vi "add filepath.vi"(6 "priority (F)":bool, 8 "error in (no error)":errorcluster, 10 "filepath":path, 11 "ComicVine_manager in":refnum<class "ComicVine_manager.lvclass">) -> (0 "error out":errorcluster, 3 "ComicVine_manager out":refnum<class "ComicVine_manager.lvclass">)   [LabVIEW 2024, in "ComicVine_manager.lvclass"]
uses:
  ComicVine_manager.lvclass
  ComicVine_manager.lvclass/ComicVine_manager.ctl
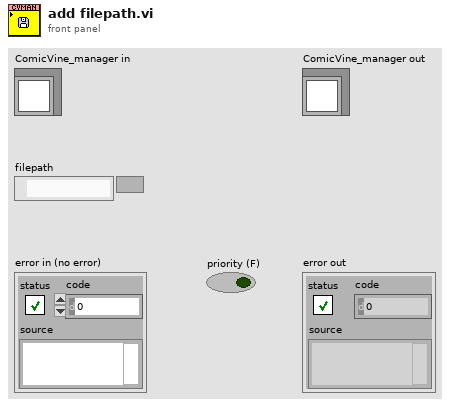
[diagram p1: front panel]
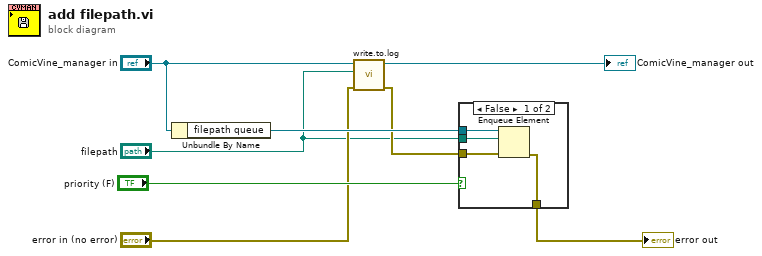
[diagram p0: block diagram]
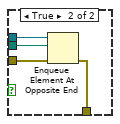
[diagram p2: hidden frame]
diagram:
  n1 = Unbundle By Name("ComicVine_manager in") -> ("filepath queue"=w8:refnum<queue>)
  n2 = call "write.to.log"("error in (no error)"="error in (no error)", "new path"="filepath", "ComicVine_manager in"="ComicVine_manager in") -> ("error out"=w3:errorcluster, "ComicVine_manager out"=→"ComicVine_manager out":refnum<class "ComicVine_manager.lvclass">)  [unwired: 7 in]
  n3 = case shown="False" "priority (F)" {
    tunnel: w8 -> [w12 w16]
    tunnel: [w11 w14] -> w7
    tunnel: "filepath" -> [w10 w15]
    tunnel: w3 -> [w9 w13]
    frame False {
      n4 = Enqueue Element(queue=w12, element=w10, error in (no error)=w9) -> (error out=w11:errorcluster)  [unwired: 1 in, 2 out]
    }
    frame True {
      n5 = Enqueue Element At Opposite End(queue=w16, element=w15, error in (no error)=w13) -> (error out=w14:errorcluster)  [unwired: 1 in, 2 out]
    }
  }
  "error out" <- w7
